vi "maintenance_check.vi"(8 "Error in (no error)":errorcluster, 9 "iteration":i32, 10 "number":i32, 11 "Connection In":refnum<k7>) -> (0 "Error out":errorcluster, 1 "Durée de vie du Courroie":string, 2 "Nombre d'heure de marche H":string, 3 "Connection Out":refnum<k7>, 4 "Nombre d'heure de marche C":string, 5 "Durée de vie du huile":string, 6 "Derniére date de changement  C":string, 7 "Derniére date de changement  H":string)   [LabVIEW 2019]
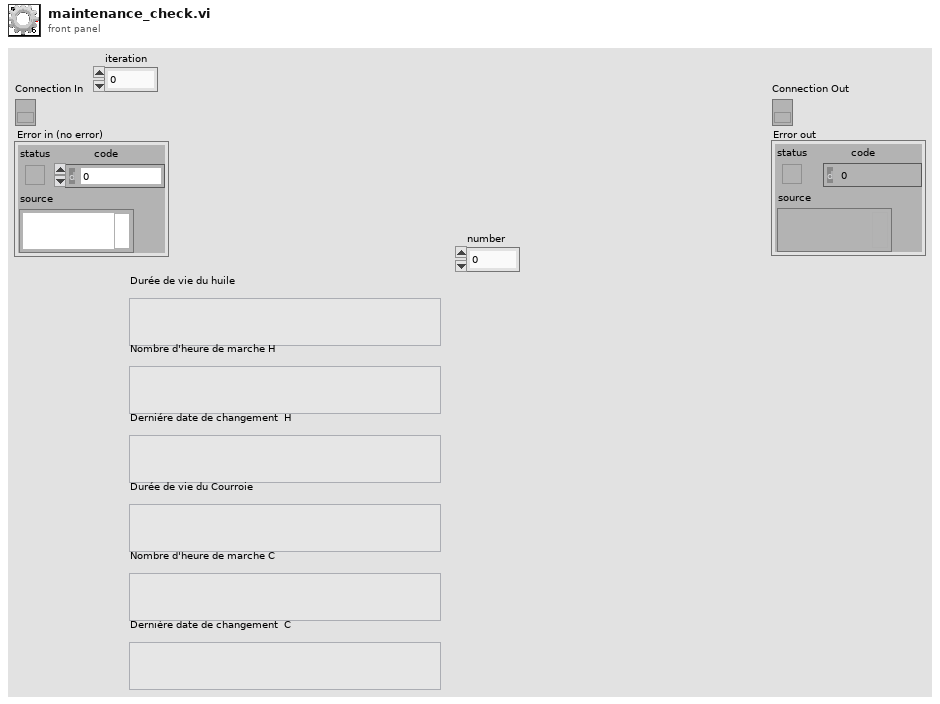
[diagram p1: front panel]
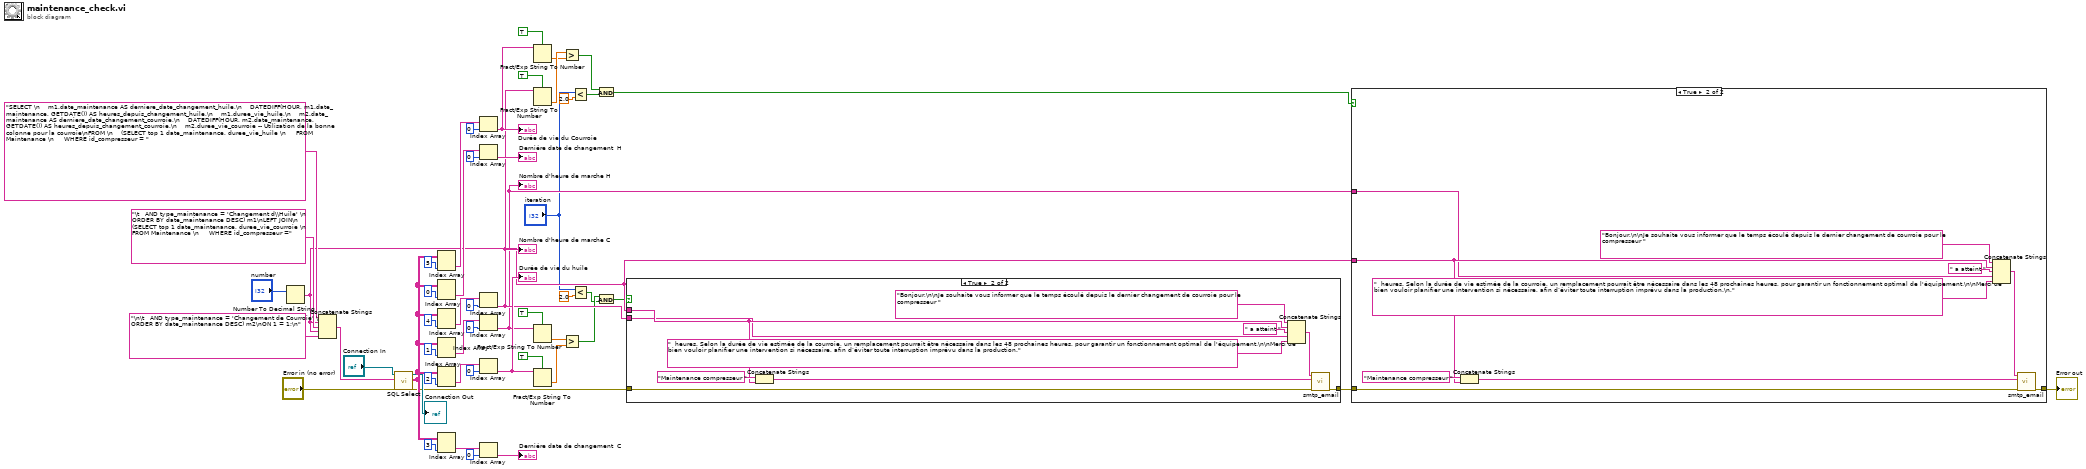
[diagram p0: block diagram]
diagram:
  n1 = Number To Decimal String(number="number") -> (decimal integer string=w14:string)  [unwired: 1 in]
  n2 = Concatenate Strings("SELECT \n    m1.date_maintenance AS derniere_date_changement_huile,\n    DATEDIFF(HOUR, m1.date_maintenance, GETDATE()) AS heures_depuis_changement_huile,\n    m1.duree_vie_huile,\n    m2.date_maintenance AS derniere_date_changement_courroie,\n    DATEDIFF(HOUR, m2.date_maintenance, GETDATE()) AS heures_depuis_changement_courroie,\n    m2.duree_vie_courroie -- Utilisation de la bonne colonne pour la courroie\nFROM \n    (SELECT top 1 date_maintenance, duree_vie_huile \n     FROM Maintenance \n     WHERE id_compresseur = ", w14, "\t   AND type_maintenance = 'Changement d\\Huile' \n     ORDER BY date_maintenance DESC) m1\nLEFT JOIN\n    (SELECT top 1 date_maintenance, duree_vie_courroie \n     FROM Maintenance \n     WHERE id_compresseur =" ("string"), w14, "\n\t   AND type_maintenance = 'Changement de Courroie' \n     ORDER BY date_maintenance DESC) m2\nON 1 = 1;\n" ("string")) -> (w44:string)
  n3 = call <vilib>:"SQL Select.vi"("Connection In"="Connection In", "SQL Query"=w44, "Error in (no error)"="Error in (no error)") -> ("Connection Out"=→"Connection Out":refnum<k7>, "Data"=w30:string[][], "Error out"=w12:errorcluster)  [unwired: 14 in]
  n4 = Index Array(array=w30, index (col)=5 ("disabled index (col)")) -> (element=w38:string[])  [unwired: 1 in]
  n5 = Index Array(array=w30, index (col)=0 ("disabled index (col)")) -> (element=w53:string[])  [unwired: 1 in]
  n6 = Index Array(array=w30, index (col)=4 ("disabled index (col)")) -> (element=w35:string[])  [unwired: 1 in]
  n7 = Index Array(array=w30, index (col)=1 ("disabled index (col)")) -> (element=w50:string[])  [unwired: 1 in]
  n8 = Index Array(array=w30, index (col)=2 ("disabled index (col)")) -> (element=w47:string[])  [unwired: 1 in]
  n9 = Index Array(array=w30, index (col)=3 ("disabled index (col)")) -> (element=w32:string[])  [unwired: 1 in]
  n10 = Index Array(array=w38, index=0) -> (element=w16:string)
  "Durée de vie du Courroie" <- w16
  n11 = Index Array(array=w53, index=0) -> (element=→"Derniére date de changement  H":string)
  n12 = Index Array(array=w35, index=0) -> (element=w15:string)
  "Nombre d'heure de marche C" <- w15
  n13 = Index Array(array=w50, index=0) -> (element=w13:string)
  "Nombre d'heure de marche H" <- w13
  n14 = Index Array(array=w47, index=0) -> (element=w23:string)
  "Durée de vie du huile" <- w23
  n15 = Index Array(array=w32, index=0) -> (element=→"Derniére date de changement  C":string)
  n16 = Fract/Exp String To Number(use system decimal point (T)=TRUE, string=w16) -> (number=w18:dbl)  [unwired: 2 in, 1 out]
  n17 = Fract/Exp String To Number(use system decimal point (T)=TRUE, string=w15) -> (number=w19:dbl)  [unwired: 2 in, 1 out]
  n18 = Fract/Exp String To Number(use system decimal point (T)=TRUE, string=w13) -> (number=w24:dbl)  [unwired: 2 in, 1 out]
  n19 = Fract/Exp String To Number(use system decimal point (T)=TRUE, string=w23) -> (number=w22:dbl)  [unwired: 2 in, 1 out]
  n20 = Greater?(x=w19, y=w18) -> (0:w2:bool)
  n21 = Greater?(x=w24, y=w22) -> (0:w8:bool)
  n22 = Less?(x="iteration", y=2.0) -> (x < y?=w4:bool)
  n23 = Less?(x="iteration", y=2.0) -> (x < y?=w7:bool)
  n24 = And(x=w2, y=w4) -> (x .and. y?=w1:bool)
  n25 = And(x=w8, y=w7) -> (x .and. y?=w6:bool)
  n26 = case shown="True" w6 {
    tunnel: w12 -> [w55 w65]
    tunnel: [w55 w64] -> w11
    tunnel: w14 -> [_ w60]
    tunnel: w15 -> [_ w59]
    frame False {
    }
    frame True {
      n27 = Concatenate Strings("Maintenance compresseur " ("string"), w60) -> (w62:string)
      n28 = Concatenate Strings("Bonjour,\n\nJe souhaite vous informer que le temps écoulé depuis le dernier changement de courroie pour le compresseur " ("string"), w60, " a atteint " ("string"), w59, "  heures. Selon la durée de vie estimée de la courroie, un remplacement pourrait être nécessaire dans les 48 prochaines heures, pour garantir un fonctionnement optimal de l'équipement.\n\nMerci de bien vouloir planifier une intervention si nécessaire, afin d’éviter toute interruption imprévu dans la production." ("string")) -> (w56:string)
      n29 = call "smtp_email.vi"("error in (no error)"=w65, "subject"=w62, "plain text message"=w56) -> ("error out"=w64:errorcluster)  [unwired: 7 in, 1 out]
    }
  }
  n30 = case shown="True" w1 {
    tunnel: w11 -> [w66 w67]
    tunnel: [w66 w76] -> w10
    tunnel: w14 -> [_ w72]
    tunnel: w13 -> [_ w71]
    frame False {
    }
    frame True {
      n31 = Concatenate Strings("Maintenance compresseur " ("string"), w72) -> (w74:string)
      n32 = Concatenate Strings("Bonjour,\n\nJe souhaite vous informer que le temps écoulé depuis le dernier changement de courroie pour le compresseur " ("string"), w72, " a atteint " ("string"), w71, "  heures. Selon la durée de vie estimée de la courroie, un remplacement pourrait être nécessaire dans les 48 prochaines heures, pour garantir un fonctionnement optimal de l'équipement.\n\nMerci de bien vouloir planifier une intervention si nécessaire, afin d’éviter toute interruption imprévu dans la production.\n," ("string")) -> (w68:string)
      n33 = call "smtp_email.vi"("error in (no error)"=w67, "subject"=w74, "plain text message"=w68) -> ("error out"=w76:errorcluster)  [unwired: 7 in, 1 out]
    }
  }
  "Error out" <- w10
